vi "vms_putSample_M1M3.vi"(8 "error in (no error)":errorcluster, 11 "M1M3_Ctl":T1) -> (0 "error out":errorcluster, 2 "function return":i32, 3 "M1M3_Ctl out":T1)   [LabVIEW 2016, in "SALLV_vms.lvlib"]
doc: "int vms_shm_putSample_M1M3LV(vms_M1M3LV *M1M3_Ctl );"
uses:
  SALLV_vms.lvlib
  DataTypes/M1M3.ctl
  SALLV_vms.so
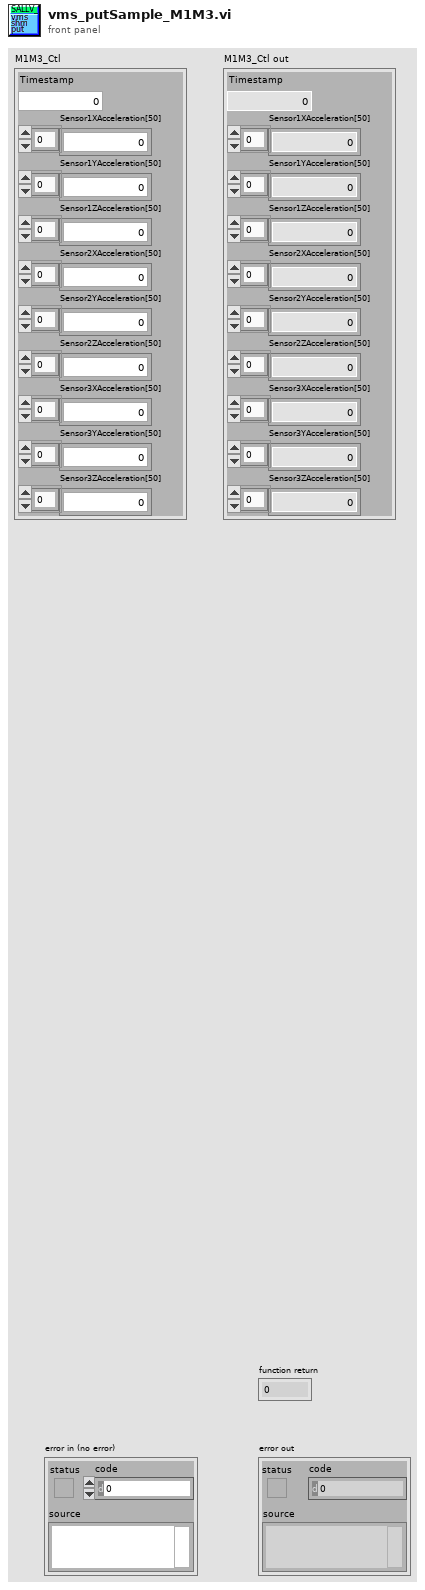
[diagram p1: front panel]
types:
  T1 = typedef "SALLV_vms.lvlib/M1M3.ctl" = cluster{"Timestamp":dbl, "Sensor1XAcceleration[50]":dbl[], "Sensor1YAcceleration[50]":dbl[], "Sensor1ZAcceleration[50]":dbl[], "Sensor2XAcceleration[50]":dbl[], "Sensor2YAcceleration[50]":dbl[], "Sensor2ZAcceleration[50]":dbl[], "Sensor3XAcceleration[50]":dbl[], "Sensor3YAcceleration[50]":dbl[], "Sensor3ZAcceleration[50]":dbl[]}
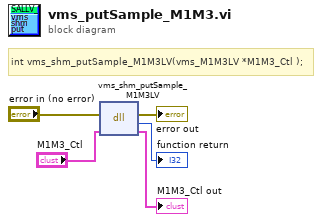
[diagram p0: block diagram]
diagram:
  # "int vms_shm_putSample_M1M3LV(vms_M1M3LV *M1M3_Ctl );"
  n1 = dll-call lib="opt/CODE/SALLV_vms/SALLV_vms.*" fn="vms_shm_putSample_M1M3LV"(error in="error in (no error)", "M1M3_Ctl"="M1M3_Ctl") -> (error out=→"error out":errorcluster, →"function return":i32, "M1M3_Ctl"=→"M1M3_Ctl out":T1)  [unwired: 2 in, 1 out]
